vi "create channels for testing.vi"() -> (0 "error out":errorcluster, 1 "names":string[](array[string]), 2 "chans":refnum<class "TBM channel.lvclass">[](array[class]), 3 "Scan Engine configuration out":refnum<class "Scan Engine configuration.lvclass">, 4 "usec scan period":u32=10000)   [LabVIEW 2013, in "scan engine tests.lvlib"]
uses:
  scan engine tests.lvlib
  configuration/Scan Engine configuration.lvclass
  <vilib>/NI/Tag Bus Module Framework/channel/TBM channel.lvclass
  <vilib>/NI/Tag Bus Module Framework/channel/channel classification.ctl
  <vilib>/NI/Tag Bus Module Framework/root configuration/TBM configuration.lvclass
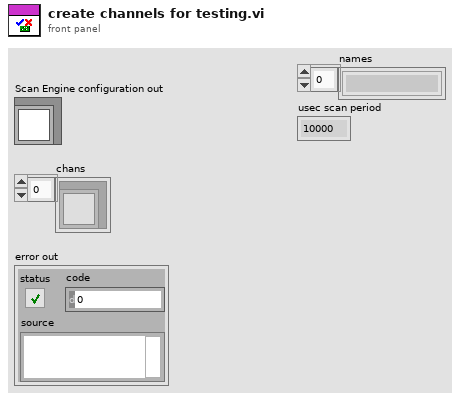
[diagram p1: front panel]
types:
  T1 = typedef "TBM channel.lvclass/channel classification.ctl" = enum16{"input data", "output data", "processing parameter", "processing result"}
  T2 = typedef "tag bus.lvlib/tag descriptor.lvclass/Data Type.ctl" = enum16{"Double", "Single", "I64", "I32", "I16", "I8", "U64", "U32", "U16", "U8", "Boolean", "String", "Array of Double", "Array of Single", "Array of I64", "Array of I32", "Array of I16", "Array of I8", "Array of U64", "Array of U32", "Array of U16", "Array of U8", "Array of Boolean", "Array of String"}
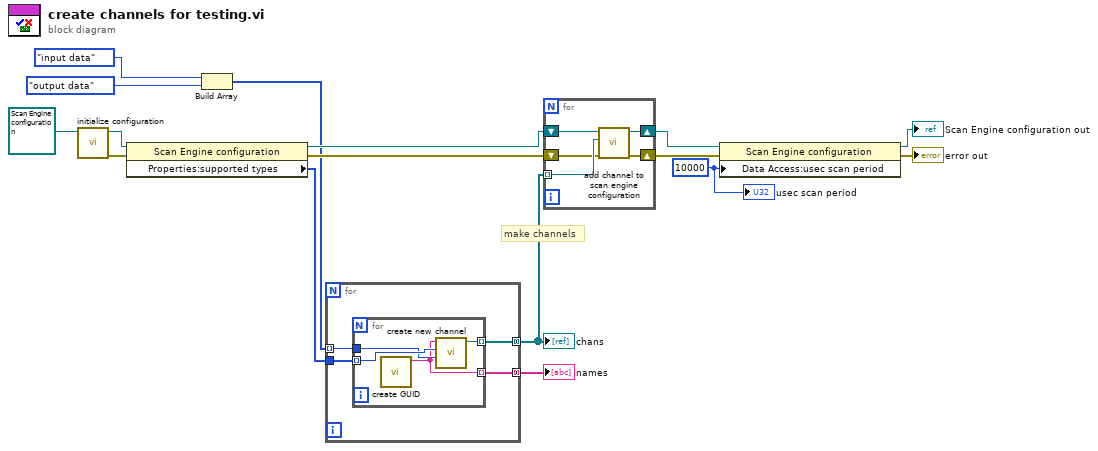
[diagram p0: block diagram]
diagram:
  w1 = u32 10000 ("usec scan period")
  # "make channels"
  n1 = call-dynamic "initialize configuration.vi"("configuration in"=refnum<class "Scan Engine configuration.lvclass"> refnum ("Scan Engine configuration")) -> ("error out"=w14:errorcluster, "configuration out"=w13:refnum<class "Scan Engine configuration.lvclass">)  [unwired: 8 in, 1 out]
  n2 = property class="Scan Engine configuration"(reference=w13, error in=w14) -> (reference out=w11:refnum<class "Scan Engine configuration.lvclass">, error out=w15:errorcluster, "Properties:supported types"=w9:T2[])
  n3 = Build Array(channel_classification."input data" ("channel classification"), channel_classification."output data" ("channel classification")) -> (w8:T1[])
  n4 = for {
    tunnel: w8 -> [w20] mode=indexing
    tunnel: [w18] -> w12 mode=concatenating
    tunnel: w9 -> [w19]
    tunnel: [w17] -> w5 mode=concatenating
    n5 = for {
      tunnel: w20 -> [w22]
      tunnel: [w24] -> w18 mode=indexing
      tunnel: w19 -> [w23] mode=indexing
      tunnel: [w21] -> w17 mode=indexing
      n6 = call <vilib>:"create GUID.vi"() -> ("uuid"=w21:string)  [unwired: 11 in]
      n7 = call <vilib>:"create new channel.vi"("channel classification"=w22, "data type"=w23, "channel name"=w21) -> ("channel"=w24:refnum<class "TBM channel.lvclass">)  [unwired: 8 in]
    }
  }
  "chans" <- w12
  "names" <- w5
  n8 = for {
    tunnel: w12 -> [w27] mode=indexing
    shift-right: [w28] -> w3
    shift-left: w11 -> [w29]
    shift-right: [w25] -> w16
    shift-left: w15 -> [w26]
    n9 = call "add channel to scan engine configuration.vi"("error in"=w26, "channel"=w27, "Scan Engine configuration in"=w29) -> ("error out"=w25:errorcluster, "Scan Engine configuration out"=w28:refnum<class "Scan Engine configuration.lvclass">)  [unwired: 7 in]
  }
  n10 = property class="Scan Engine configuration"(reference=w3, error in=w16, "Data Access:usec scan period"=w1) -> (reference out=→"Scan Engine configuration out":refnum<class "Scan Engine configuration.lvclass">, error out=→"error out":errorcluster)
  "usec scan period" <- w1
